vi "Begin.vi"(8 "error in (no error)":errorcluster, 11 "One Driver in":refnum<class "One Driver.lvclass">) -> (0 "error out":errorcluster, 3 "One Driver out":refnum<class "One Driver.lvclass">)   [LabVIEW 2018, in "Joysticks.lvlib" / "One Driver.lvclass"]
doc: "This VI is used to open the joystick control references."
uses:
  One Driver.lvclass
  <vilib>/Rock Robotics/WPI/Joystick/WPI_JoystickDeviceEnum.ctl
  One Driver.lvclass/One Driver.ctl
  Joysticks.lvclass
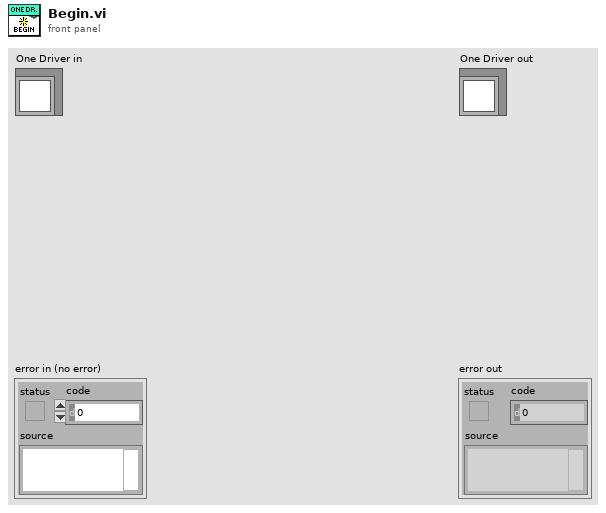
[diagram p1: front panel]
types:
  T1 = typedef "WPI_JoystickDeviceEnum.ctl" = enum16{"USB 0", "USB 1", "USB 2", "USB 3", "USB 4", "USB 5"}
  T2 = typedef "WPI_JoystickDevRef.ctl" = cluster{"Device":T1}
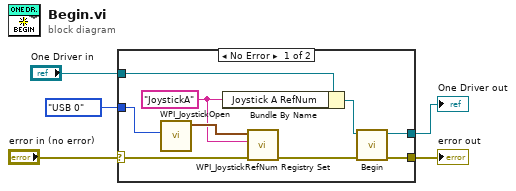
[diagram p0: block diagram]
diagram:
  n1 = case shown="No Error" "error in (no error)" {
    selector: "error in (no error)" -> [w10 w16]
    tunnel: [w14 w16] -> w5
    tunnel: [w13 w15] -> w4
    tunnel: "One Driver in" -> [w12 w15]
    tunnel: WPI_JoystickDeviceEnum."USB 0" ("JoystickDevice") -> [w8 _]
    frame No Error {
      w6 = "JoystickA" ("Joystick A RefNum")
      n2 = call <vilib>:"WPI_JoystickOpen.vi"("JoystickDevice"=w8) -> ("JoystickDevRef"=w11:T2)  [unwired: 10 in]
      n3 = Bundle By Name(cluster=w12, "Joystick A RefNum"=w6) -> (w7:refnum<class "One Driver.lvclass">)
      n4 = call <vilib>:"WPI_JoystickRefNum Registry Set.vi"("error in (no error)"=w10, "refnum name"=w6, "JoystickDevRef"=w11) -> ("error out"=w9:errorcluster)  [unwired: 7 in, 1 out]
      n5 = call-parent "Begin.vi"("error in (no error)"=w9, "Joysticks in"=w7) -> ("error out"=w14:errorcluster, "Joysticks out"=w13:refnum<class "One Driver.lvclass">)  [unwired: 8 in]
    }
    frame Error {
    }
  }
  "error out" <- w5
  "One Driver out" <- w4
